vi "Memory Test.vi"() -> ()   [LabVIEW 2015]
doc: "Tests Modbus Server by writing to random memory locations, reading back and comparing data."
uses:
  PL Modbus Client.lvclass
panel:
  out "command":string
  in  "number of iterations":u32=100
  out "progress":dbl(slide) scale=0.0..1.0
  out "memory readback error":bool
  in  "number of holding registers":u16=50
  in  "number of coils":u16=800
  in  "interface":enum32{"serial", "TCP"}(tab)
  in  "serial settings":T1={"port"="", "protocol"=enum."RTU", "address"=1, "baud rate"=9600, "data bits"=8, "parity"=2, "stop bits"=10, "flow control"=0} {"flow control" items=["None", "XON/XOFF", "RTS/CTS", "XON/XOFF & RTS/CTS", "DTR/DSR", "XON/XOFF & DTR/DSR"]; "stop bits" items=["1.0"=10, "1.5"=15, "2.0"=20]; "parity" items=["None", "Odd", "Even", "Mark", "Space"]}
  in  "TCP settings":T2={"ip address"="192.168.1.1", "port"=502, "station address"=255}
  in  "timeout, ms":u32=300
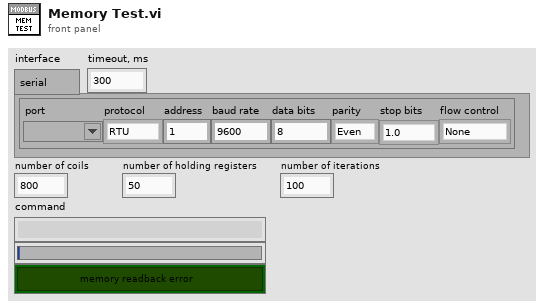
[diagram p1: front panel]
types:
  T1 = cluster{"port":refnum<visa-resource-name>, "protocol":enum16{"RTU", "ASCII"}, "address":u8, "baud rate":u32, "data bits":u16, "parity":u16, "stop bits":u16, "flow control":u16}
  T2 = cluster{"ip address":string, "port":u16, "station address":u8}
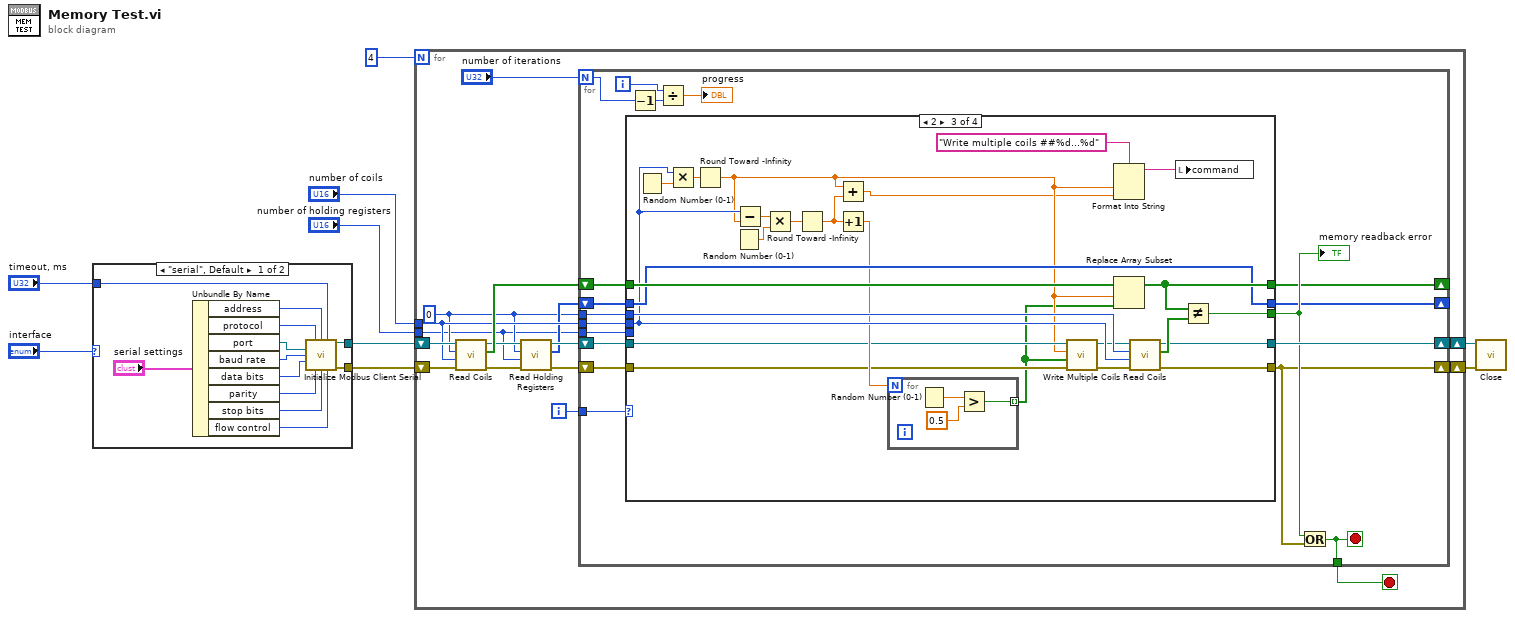
[diagram p0: block diagram]
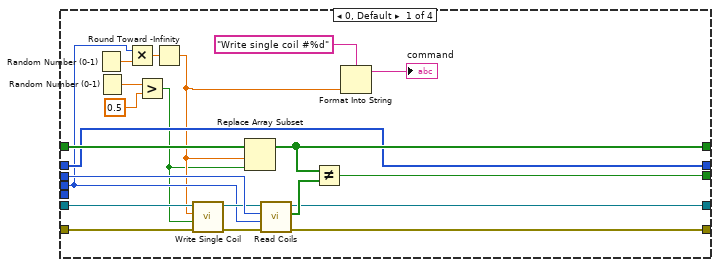
[diagram p2: hidden frame]
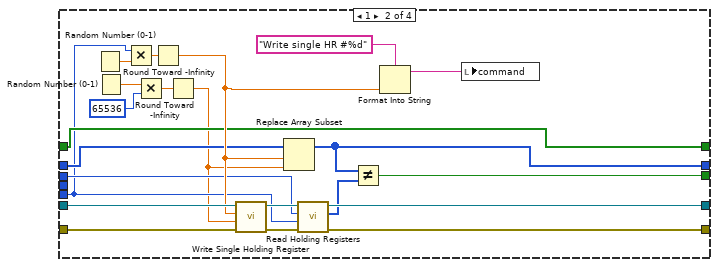
[diagram p3: hidden frame]
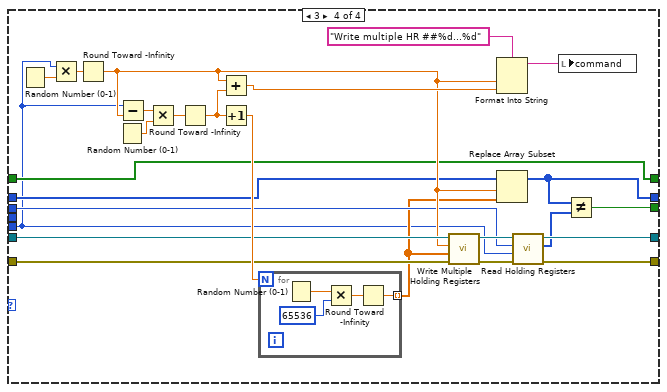
[diagram p4: hidden frame]
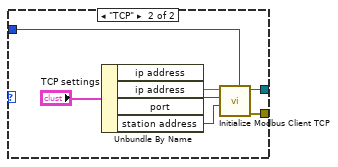
[diagram p5: hidden frame]
diagram:
  n1 = case shown="\"serial\", Default" "interface" {
    tunnel: [w21 w26] -> w1
    tunnel: [w20 w25] -> w2
    tunnel: "timeout, ms" -> [w12 w22]
    frame "serial", Default {
      n2 = Unbundle By Name("serial settings") -> ("address"=w11:u8, "protocol"=w10:enum16{"RTU", "ASCII"}, "port"=w19:refnum<visa-resource-name>, "baud rate"=w14:u32, "data bits"=w15:u16, "parity"=w16:u16, "stop bits"=w17:u16, "flow control"=w18:u16)
      n3 = call "Initialize Modbus Client Serial.vi"("protocol (RTU)"=w10, "station address (1)"=w11, "timeout, ms (300)"=w12, "port"=w19, "baud rate (9600)"=w14, "data bits (8)"=w15, "parity (even)"=w16, "stop bits (1.0)"=w17, "flow control (none)"=w18) -> ("MODBUS out"=w21:refnum<class "PL Modbus Client.lvclass">, "error out"=w20:errorcluster)  [unwired: 5 in]
    }
    frame "TCP" {
      n4 = Unbundle By Name("TCP settings") -> ("ip address"=w28:string, "port"=w27:u16, "station address"=w23:u8)  [unwired: 1 out]
      n5 = call "Initialize Modbus Client TCP.vi"("timeout, ms (300)"=w22, "station address (255)"=w23, "port (502)"=w27, "ip address"=w28) -> ("error out"=w25:errorcluster, "MODBUS out"=w26:refnum<class "PL Modbus Client.lvclass">)  [unwired: 6 in]
    }
  }
  n6 = for {
    N: 4 -> [_]
    shift-right: [w42] -> w6
    shift-left: w1 -> [w40]
    shift-right: [w43] -> w5
    shift-left: w2 -> [w39]
    tunnel: "number of coils" -> [w37]
    tunnel: "number of holding registers" -> [w30]
    i -> [w44]
    stop <- w41 stop-if-true
    w31 = u16 0 ("first address")
    n7 = call "Read Coils.vi"("error in (no error)"=w39, "number of coils"=w37, "address"=w31, "MODBUS in"=w40) -> ("error out"=w33:errorcluster, "values"=w38:bool[], "MODBUS out"=w36:refnum<class "PL Modbus Client.lvclass">)  [unwired: 5 in]
    n8 = call "Read Holding Registers.vi"("error in (no error)"=w33, "number of holding registers"=w30, "address"=w31, "MODBUS in"=w36) -> ("error out"=w34:errorcluster, "values"=w32:u16[], "MODBUS out"=w35:refnum<class "PL Modbus Client.lvclass">)  [unwired: 5 in]
    n9 = for {
      N: "number of iterations" -> [w47]
      shift-right: [w56] -> w42
      shift-left: w35 -> [w59]
      tunnel: w44 -> [w60]
      shift-right: [w52] -> _
      shift-left: w38 -> [w62]
      shift-right: [w51] -> _
      shift-left: w32 -> [w61]
      tunnel: w31 -> [w57]
      shift-right: [w54] -> w43
      shift-left: w34 -> [w58]
      tunnel: [w53] -> w41
      tunnel: w37 -> [w50]
      tunnel: w30 -> [w49]
      i -> [w48]
      stop <- w53 stop-if-true
      n10 = case shown="2" w60 {
        tunnel: w62 -> [w74 w89 w127 w142]
        tunnel: w61 -> [w68 w91 w121 w144]
        tunnel: w59 -> [w83 w98 w114 w146]
        tunnel: w58 -> [w82 w99 w113 w147]
        tunnel: w57 -> [w77 w88 w128 w136]
        tunnel: [w72 w96 w125 w138] -> w56
        tunnel: [w71 w95 w124 w140] -> w54
        tunnel: [w70 w102 w123 w156] -> w55
        tunnel: [w69 w89 w122 w142] -> w52
        tunnel: [w68 w90 w121 w143] -> w51
        tunnel: w50 -> [w67 _ w118 _]
        tunnel: w49 -> [_ w86 _ w134]
        frame 0, Default {
          n11 = Random Number (0-1)() -> (number: 0 to 1=w81:dbl)
          n12 = Random Number (0-1)() -> (number: 0 to 1=w79:dbl)
          n13 = Multiply(x=w67, y=w81) -> (x*y=w80:dbl)
          n14 = Greater?(x=w79, y=0.5) -> (0:w64:bool)
          n15 = Round Toward -Infinity(1:w80) -> (0:w65:dbl)
          n16 = call "Write Single Coil.vi"("error in (no error)"=w82, "value"=w64, "address"=w65, "MODBUS in"=w83) -> ("error out"=w75:errorcluster, "MODBUS out"=w76:refnum<class "PL Modbus Client.lvclass">)  [unwired: 6 in]
          n17 = Replace Array Subset(array=w74, new element=w64, index=w65) -> (w69:bool[])
          n18 = call "Read Coils.vi"("error in (no error)"=w75, "number of coils"=w67, "address"=w77, "MODBUS in"=w76) -> ("error out"=w71:errorcluster, "values"=w73:bool[], "MODBUS out"=w72:refnum<class "PL Modbus Client.lvclass">)  [unwired: 5 in]
          n19 = Not Equal?(x=w69, y=w73) -> (x != y?=w70:bool)
          n20 = Format Into String(format string="Write single coil #%d", w65) -> (resulting string=→"command":string)  [unwired: 2 in, 1 out]
        }
        frame 1 {
          n21 = Random Number (0-1)() -> (number: 0 to 1=w105:dbl)
          n22 = Random Number (0-1)() -> (number: 0 to 1=w103:dbl)
          n23 = Multiply(x=w86, y=w105) -> (x*y=w104:dbl)
          n24 = Multiply(x=w103, y=u32 65536) -> (x*y=w85:dbl)
          n25 = Round Toward -Infinity(1:w104) -> (0:w97:dbl)
          n26 = Round Toward -Infinity(1:w85) -> (0:w84:dbl)
          n27 = call "Write Single Holding Register.vi"("error in (no error)"=w99, "value"=w84, "address"=w97, "MODBUS in"=w98) -> ("error out"=w94:errorcluster, "MODBUS out"=w93:refnum<class "PL Modbus Client.lvclass">)  [unwired: 6 in]
          n28 = Replace Array Subset(array=w91, new element=w84, index=w97) -> (w90:u16[])
          n29 = call "Read Holding Registers.vi"("error in (no error)"=w94, "number of holding registers"=w86, "address"=w88, "MODBUS in"=w93) -> ("error out"=w95:errorcluster, "values"=w92:u16[], "MODBUS out"=w96:refnum<class "PL Modbus Client.lvclass">)  [unwired: 5 in]
          n30 = Not Equal?(x=w90, y=w92) -> (x != y?=w102:bool)
          n31 = Format Into String(format string="Write single HR #%d", w97) -> (resulting string=w87:string)  [unwired: 2 in, 1 out]
          n32 = local write "command"(w87) -> ()
        }
        frame 2 {
          n33 = Random Number (0-1)() -> (number: 0 to 1=w130:dbl)
          n34 = Multiply(x=w118, y=w130) -> (x*y=w129:dbl)
          n35 = Round Toward -Infinity(1:w129) -> (0:w110:dbl)
          n36 = Random Number (0-1)() -> (number: 0 to 1=w117:dbl)
          n37 = Subtract(x=w118, y=w110) -> (x-y=w116:dbl)
          n38 = Multiply(x=w116, y=w117) -> (x*y=w106:dbl)
          n39 = Round Toward -Infinity(1:w106) -> (0:w109:dbl)
          n40 = Add(x=w110, y=w109) -> (x+y=w108:dbl)
          n41 = Increment(x=w109) -> (x+1=w115:dbl)
          n42 = for {
            N: w115 -> [_]
            tunnel: [w131] -> w107 mode=indexing
            n43 = Random Number (0-1)() -> (number: 0 to 1=w133:dbl)
            n44 = Greater?(x=w133, y=0.5) -> (0:w131:bool)
          }
          n45 = call "Write Multiple Coils.vi"("error in (no error)"=w113, "values"=w107, "address"=w110, "MODBUS in"=w114) -> ("error out"=w111:errorcluster, "MODBUS out"=w112:refnum<class "PL Modbus Client.lvclass">)  [unwired: 6 in]
          n46 = Format Into String(format string="Write multiple coils ##%d...%d", w110, w108) -> (resulting string=w119:string)  [unwired: 2 in, 1 out]
          n47 = Replace Array Subset(array=w127, new element=w107, index=w110) -> (w122:bool[])
          n48 = call "Read Coils.vi"("error in (no error)"=w111, "number of coils"=w118, "address"=w128, "MODBUS in"=w112) -> ("error out"=w124:errorcluster, "values"=w126:bool[], "MODBUS out"=w125:refnum<class "PL Modbus Client.lvclass">)  [unwired: 5 in]
          n49 = local write "command"(w119) -> ()
          n50 = Not Equal?(x=w122, y=w126) -> (x != y?=w123:bool)
        }
        frame 3 {
          n51 = Random Number (0-1)() -> (number: 0 to 1=w158:dbl)
          n52 = Multiply(x=w134, y=w158) -> (x*y=w157:dbl)
          n53 = Round Toward -Infinity(1:w157) -> (0:w145:dbl)
          n54 = Random Number (0-1)() -> (number: 0 to 1=w153:dbl)
          n55 = Subtract(x=w134, y=w145) -> (x-y=w151:dbl)
          n56 = Multiply(x=w151, y=w153) -> (x*y=w152:dbl)
          n57 = Round Toward -Infinity(1:w152) -> (0:w149:dbl)
          n58 = Add(x=w145, y=w149) -> (x+y=w148:dbl)
          n59 = Increment(x=w149) -> (x+1=w150:dbl)
          n60 = for {
            N: w150 -> [_]
            tunnel: [w159] -> w135 mode=indexing
            n61 = Random Number (0-1)() -> (number: 0 to 1=w160:dbl)
            n62 = Multiply(x=w160, y=u32 65536) -> (x*y=w162:dbl)
            n63 = Round Toward -Infinity(1:w162) -> (0:w159:dbl)
          }
          n64 = call "Write Multiple Holding Registers.vi"("error in (no error)"=w147, "values"=w135, "address"=w145, "MODBUS in"=w146) -> ("error out"=w139:errorcluster, "MODBUS out"=w141:refnum<class "PL Modbus Client.lvclass">)  [unwired: 6 in]
          n65 = Format Into String(format string="Write multiple HR ##%d...%d", w145, w148) -> (resulting string=w154:string)  [unwired: 2 in, 1 out]
          n66 = Replace Array Subset(array=w144, new element=w135, index=w145) -> (w143:u16[])
          n67 = call "Read Holding Registers.vi"("error in (no error)"=w139, "number of holding registers"=w134, "address"=w136, "MODBUS in"=w141) -> ("error out"=w140:errorcluster, "values"=w137:u16[], "MODBUS out"=w138:refnum<class "PL Modbus Client.lvclass">)  [unwired: 5 in]
          n68 = local write "command"(w154) -> ()
          n69 = Not Equal?(x=w143, y=w137) -> (x != y?=w156:bool)
        }
      }
      "memory readback error" <- w55
      n70 = Decrement(x=w47) -> (x-1=w46:i32)
      n71 = Divide(x=w48, y=w46) -> (x/y=→"progress":dbl)
      n72 = Or(x=w55, y=w54) -> (x .or. y?=w53:bool)
    }
  }
  n73 = call-dynamic "Close.vi"("error in (no error)"=w5, "MODBUS in"=w6) -> ()  [unwired: 9 in, 1 out]
